vi "Create Tower.vi"(8 "error in (no error)":errorcluster, 9 "Location":T1, 10 "Tower Height":sgl, 11 "Main Scene Object":refnum<vi>) -> (0 "error out":errorcluster, 3 "Main Scene Object (out)":refnum<vi>)   [LabVIEW 2023]
doc: "Create a cone object for the tower."
uses:
  <vilib>/Utility/miscctls.llb/LV3DPointTypeDef.ctl
  <vilib>/picture/3D Picture Control/Object/Create Object (drawable).vi
  <vilib>/picture/3D Picture Control/Object/Create Object (name).vi
  <vilib>/picture/3D Picture Control/Object/Add Object (no reference).vi
  <vilib>/picture/3D Picture Control/NI_3D Picture Control.lvlib
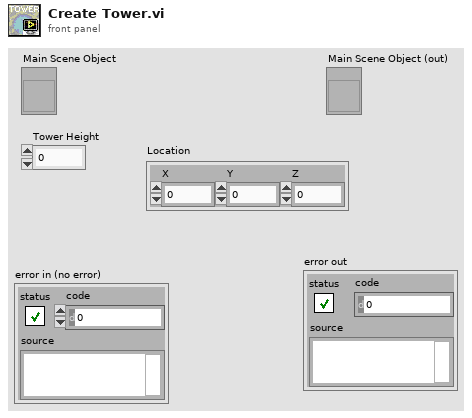
[diagram p1: front panel]
types:
  T1 = typedef "LV3DPointTypeDef.ctl" = cluster{"X":sgl, "Y":sgl, "Z":sgl}
  T2 = enum16{"Normal Bin", "Opaque Bin", "Transparent Bin"}
  T3 = enum16{"Inherit Value", "No Culling", "Cull Back Face", "Cull Front Face", "Cull Both Faces"}
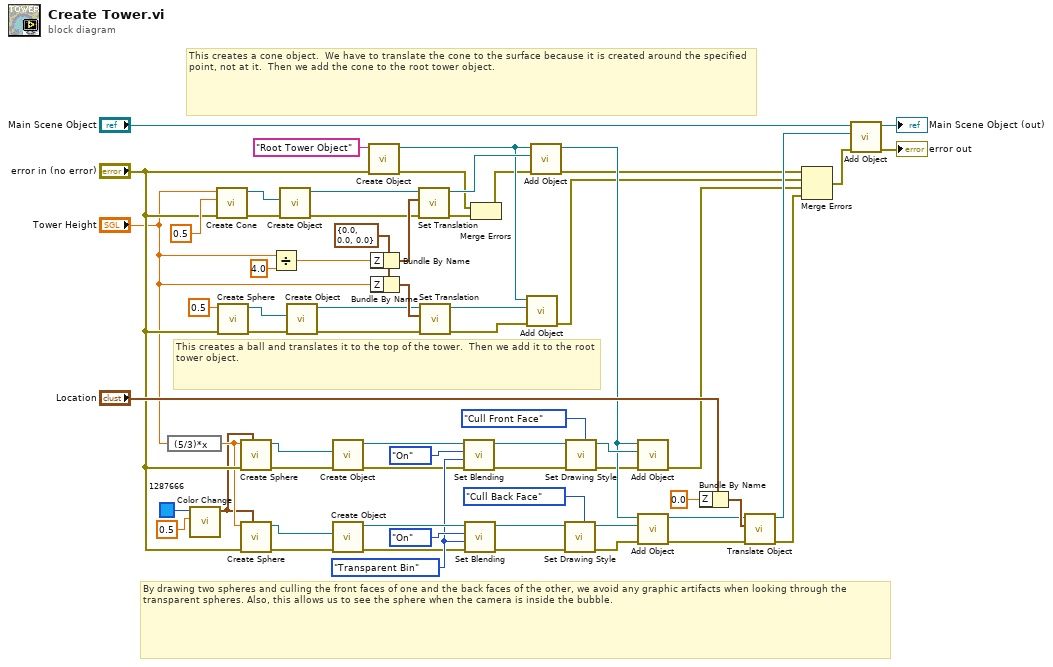
[diagram p0: block diagram]
diagram:
  w33 = T2."Transparent Bin" ("Blending:Bin")
  w57 = cluster{"X":sgl, "Y":sgl, "Z":sgl} {"X"=0.0, "Y"=0.0, "Z"=0.0} ("Translation")
  # "This creates a ball and translates it to the top of the tower.  Then we add it to the root tower object."
  # "This creates a cone object.  We have to translate the cone to the surface because it is created around the specified point, not at it.  Then we add the cone to the root tower object."
  # "By drawing two spheres and culling the front faces of one and the back faces of the other, we avoid any graphic artifacts when looking through the transparent spheres. Also, this allows us to see the sphere when the camera is inside the bubble."
  n1 = expression code="(5/3)*x"("Tower Height") -> (w2:sgl)
  n2 = call <vilib>:"Color Change.vi"("Alpha"=0.5, "Color"=u32 1287666) -> ("RGBA"=w1:cluster{"R":sgl, "G":sgl, "B":sgl, "A":sgl})  [unwired: 9 out]
  n3 = call <vilib>:"Create Cone.vi"("error in (no error)"="error in (no error)", "Radius"=sgl 0.5, "Height"="Tower Height") -> ("error out"=w44:errorcluster, "New Cone Refnum"=w53:refnum<vi>)  [unwired: 7 out]
  n4 = call <vilib>:"Create Sphere.vi"("error in (no error)"="error in (no error)", "Radius"=sgl 0.5) -> ("error out"=w46:errorcluster, "New Sphere Refnum"=w48:refnum<vi>)  [unwired: 8 out]
  n5 = call <vilib>:"Create Sphere.vi"("Color"=w1, "error in (no error)"="error in (no error)", "Radius"=w2) -> ("error out"=w24:errorcluster, "New Sphere Refnum"=w42:refnum<vi>)  [unwired: 7 out]
  n6 = call <vilib>:"Create Sphere.vi"("Color"=w1, "error in (no error)"="error in (no error)", "Radius"=w2) -> ("error out"=w20:errorcluster, "New Sphere Refnum"=w41:refnum<vi>)  [unwired: 7 out]
  n7 = Divide(x="Tower Height", y=4.0) -> (x/y=w58:dbl)
  n8 = call-poly <vilib>:"Create Object.vi"("error in (no error)"=w44, "Geometry"=w53) -> ("error out"=w43:errorcluster, "Scene:New Object"=w52:refnum<vi>)  [unwired: 8 in]
  n9 = call-poly <vilib>:"Create Object.vi"("error in (no error)"=w46, "Geometry"=w48) -> ("error out"=w45:errorcluster, "Scene:New Object"=w47:refnum<vi>)  [unwired: 8 in]
  n10 = call-poly <vilib>:"Create Object.vi"("error in (no error)"=w24, "Geometry"=w42) -> ("error out"=w23:errorcluster, "Scene:New Object"=w40:refnum<vi>)  [unwired: 8 in]
  n11 = call-poly <vilib>:"Create Object.vi"("error in (no error)"=w20, "Geometry"=w41) -> ("error out"=w19:errorcluster, "Scene:New Object"=w35:refnum<vi>)  [unwired: 8 in]
  n12 = call-poly <vilib>:"Create Object.vi"("error in (no error)"="error in (no error)", "Name"="Root Tower Object") -> ("error out"=w14:errorcluster, "Scene:New Object"=w50:refnum<vi>)  [unwired: 8 in]
  n13 = Bundle By Name(cluster=w57, "Z"=w58) -> (w60:cluster{"X":sgl, "Y":sgl, "Z":sgl})
  n14 = Bundle By Name(cluster=w57, "Z"="Tower Height") -> (w61:cluster{"X":sgl, "Y":sgl, "Z":sgl})
  n15 = call <vilib>:"Set Translation.vi"("error in (no error)"=w43, "Translation"=w60, "Scene Object"=w52) -> ("error out"=w15:errorcluster, "Translated Object"=w51:refnum<vi>)  [unwired: 7 out]
  n16 = call <vilib>:"Set Translation.vi"("error in (no error)"=w45, "Translation"=w61, "Scene Object"=w47) -> ("error out"=w12:errorcluster, "Translated Object"=w49:refnum<vi>)  [unwired: 7 out]
  n17 = call <vilib>:"Set Blending.vi"("error in (no error)"=w23, "Bin"=w33, "Mode"=enum16{"Inherit Value", "Off", "On"}."On" ("Blending:Mode"), "Scene Object In"=w40) -> ("error out"=w22:errorcluster, "Scene Object Out"=w38:refnum<vi>)  [unwired: 6 in]
  n18 = call <vilib>:"Set Blending.vi"("error in (no error)"=w19, "Bin"=w33, "Mode"=enum16{"Inherit Value", "Off", "On"}."On" ("Blending:Mode"), "Scene Object In"=w35) -> ("error out"=w18:errorcluster, "Scene Object Out"=w31:refnum<vi>)  [unwired: 6 in]
  n19 = Merge Errors(w14, w15) -> (w13:errorcluster)
  n20 = call-poly <vilib>:"Add Object.vi"("error in (no error)"=w12, "New Object In"=w49, "Scene Object In"=w50) -> ("error out"=w9:errorcluster)  [unwired: 7 in, 1 out]
  n21 = call-poly <vilib>:"Add Object.vi"("error in (no error)"=w13, "New Object In"=w51, "Scene Object In"=w50) -> ("error out"=w8:errorcluster, "Scene Object Out"=w30:refnum<vi>)  [unwired: 7 in]
  n22 = call <vilib>:"Set Drawing Style.vi"("Face Culling Mode"=T3."Cull Back Face" ("Draw Style:Face Culling Mode"), "error in (no error)"=w18, "Scene Object In"=w31) -> ("error out"=w17:errorcluster, "Scene Object Out"=w29:refnum<vi>)  [unwired: 7 in]
  n23 = call <vilib>:"Set Drawing Style.vi"("Face Culling Mode"=T3."Cull Front Face" ("Draw Style:Face Culling Mode"), "error in (no error)"=w22, "Scene Object In"=w38) -> ("error out"=w21:errorcluster, "Scene Object Out"=w36:refnum<vi>)  [unwired: 7 in]
  n24 = call-poly <vilib>:"Add Object.vi"("error in (no error)"=w21, "New Object In"=w36, "Scene Object In"=w30) -> ("error out"=w11:errorcluster)  [unwired: 7 in, 1 out]
  n25 = call-poly <vilib>:"Add Object.vi"("error in (no error)"=w17, "New Object In"=w29, "Scene Object In"=w30) -> ("error out"=w16:errorcluster, "Scene Object Out"=w28:refnum<vi>)  [unwired: 7 in]
  n26 = Bundle By Name(cluster="Location", "Z"=sgl 0.0 ("Radius")) -> (w54:T1)
  n27 = call <vilib>:"Translate Object.vi"("error in (no error)"=w16, "Translation"=w54, "Scene.Object In"=w28) -> ("error out"=w10:errorcluster, "Scene.Object Out"=w26:refnum<vi>)  [unwired: 7 out]
  n28 = Merge Errors(w8, w9, w11, w10) -> (w7:errorcluster)
  n29 = call-poly <vilib>:"Add Object.vi"("error in (no error)"=w7, "New Object In"=w26, "Scene Object In"="Main Scene Object") -> ("error out"=→"error out":errorcluster, "Scene Object Out"=→"Main Scene Object (out)":refnum<vi>)  [unwired: 7 in]
